vi "Accumulate relay names.vi"(8 "error in (no error)":errorcluster, 11 "2525 in":refnum<class "2525.lvclass">) -> (0 "error out":errorcluster, 3 "2525 out":refnum<class "2525.lvclass">)   [LabVIEW 2019, in "2525.lvlib" / "2525.lvclass"]
uses:
  Library/2525.lvclass
  Library/2525.lvclass/2525.ctl
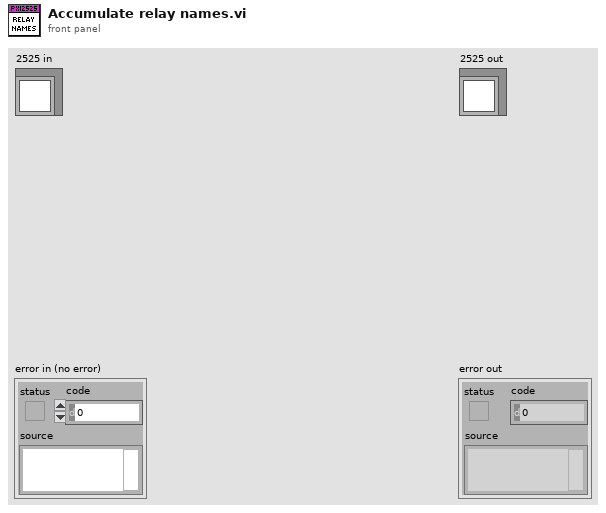
[diagram p1: front panel]
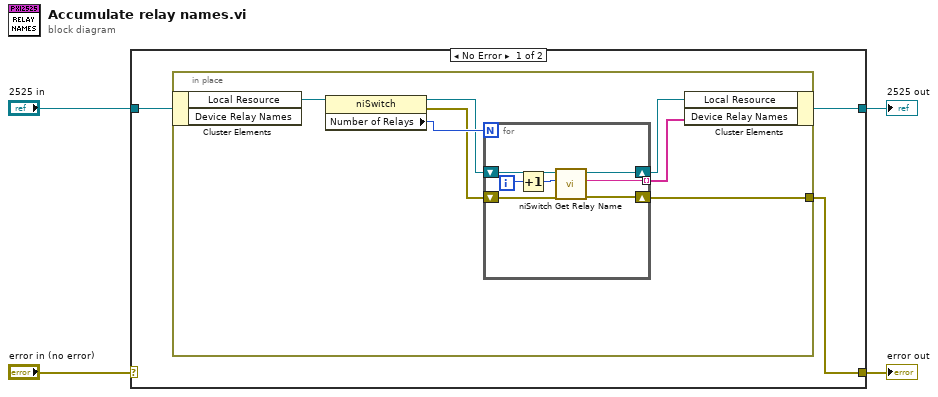
[diagram p0: block diagram]
diagram:
  n1 = case shown="No Error" "error in (no error)" {
    selector: "error in (no error)" -> [_ w23]
    tunnel: [w5 w23] -> w3
    tunnel: [w6 w22] -> w1
    tunnel: "2525 in" -> [w7 w22]
    frame No Error {
      n2 = in-place {
        in-place-border: [w8] -> w5
        n3 = in-place-cluster #1(w7) -> ("Local Resource"=w14:refnum<k15>)  [unwired: 1 out]
        n4 = property class="niSwitch"(reference=w14) -> (reference out=w12:refnum<k15>, error out=w11:errorcluster, "Number of Relays"=w13:i32)  [unwired: 1 in]
        n5 = for {
          N: w13 -> [_]
          shift-right: [w20] -> w10
          shift-left: w12 -> [w21]
          shift-right: [w17] -> w8
          shift-left: w11 -> [w16]
          tunnel: [w15] -> w9 mode=indexing
          i -> [w18]
          n6 = Increment(x=w18) -> (x+1=w19:i32)
          n7 = call <instrlib>:"niSwitch Get Relay Name.vi"("error in (no error)"=w16, "index (1)"=w19, "instrument handle"=w21) -> ("error out"=w17:errorcluster, "relay name"=w15:string, "instrument handle out"=w20:refnum<k15>)  [unwired: 6 in]
        }
        n8 = in-place-cluster #1("Local Resource"=w10, "Device Relay Names"=w9) -> (w6:refnum<class "2525.lvclass">)
      }
    }
    frame Error {
    }
  }
  "error out" <- w3
  "2525 out" <- w1
